vi "Read Input.vi"(8 "error in (no error)":errorcluster, 11 "Termination in":refnum<class "Termination.lvclass">) -> (0 "error out":errorcluster, 2 "Input":i32, 3 "Termination out":refnum<class "Termination.lvclass">)   [LabVIEW 2020, in "Termination.lvclass"]
uses:
  Termination.lvclass
  Termination.lvclass/Termination.ctl
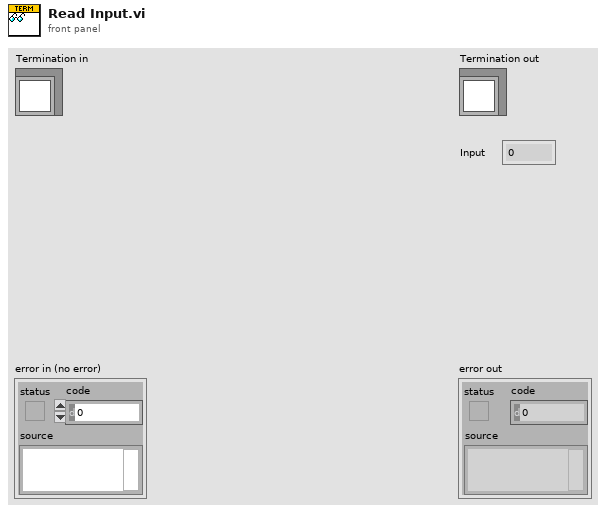
[diagram p1: front panel]
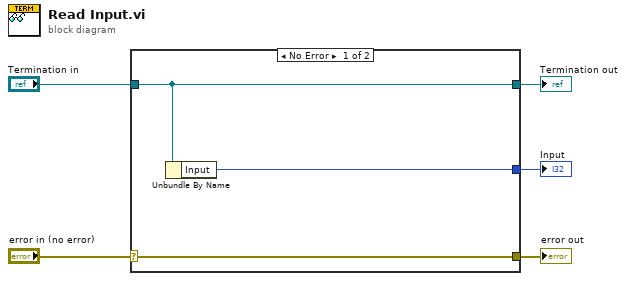
[diagram p0: block diagram]
diagram:
  n1 = case shown="No Error" "error in (no error)" {
    selector: "error in (no error)" -> [w8 w9]
    tunnel: [w8 w9] -> w4
    tunnel: [w7 w10] -> w2
    tunnel: "Termination in" -> [w7 w10]
    tunnel: [w6 _] -> w1
    frame No Error {
      n2 = Unbundle By Name(w7) -> ("Input"=w6:i32)
    }
    frame Error {
    }
  }
  "error out" <- w4
  "Termination out" <- w2
  "Input" <- w1
